vi "Map Channel.vi"(10 "Destination":refnum<k24>, 11 "Source":refnum<k24>) -> (2 "Destination Path":string, 3 "Source Path":string)   [LabVIEW 2019, in "Software Multi-Plex System Explorer.lvlib"]
uses:
  Software Multi-Plex System Explorer.lvlib
  NationalInstruments.VeriStand.SystemStorage
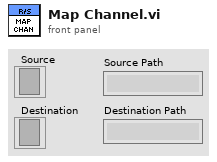
[diagram p1: front panel]
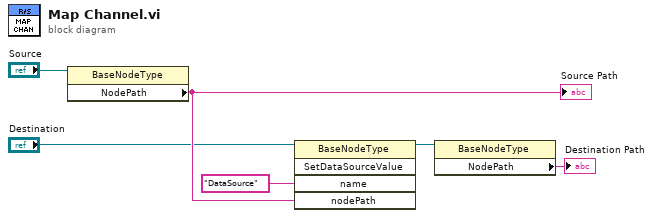
[diagram p0: block diagram]
diagram:
  n1 = property class="BaseNodeType"(reference="Source") -> ("NodePath"=w4:string)  [unwired: 1 in, 2 out]
  "Source Path" <- w4
  n2 = invoke class="BaseNodeType" method="SetDataSourceValue"(reference="Destination", "name"="DataSource", "nodePath"=w4) -> (reference out=w2:refnum<k24>)  [unwired: 2 in, 4 out]
  n3 = property class="BaseNodeType"(reference=w2) -> ("NodePath"=→"Destination Path":string)  [unwired: 1 in, 2 out]
